vi "AskListName.vi"(1 "Default name":string, 5 "error in (no error)":errorcluster) -> (17 "List":string, 18 "OK":bool, 19 "error out":errorcluster)   [LabVIEW 2022 SP3]
doc: "Displays a standard dialog box that prompts users to enter information, such as a user name and password.\n--------------------\n\nThis Express VI is configured as follows:\n\nMessage to Display to the User:Enter the name of the new list.\nThe inputs are: \nText Entry Box: List"
uses:
  <vilib>/Utility/miscctls.llb/LVSelectionTypeDef.ctl
panel:
  in  "List":string
  out "String":string="Enter the name of the new list."
  in  "Cancel":bool
  in  "OK2":bool
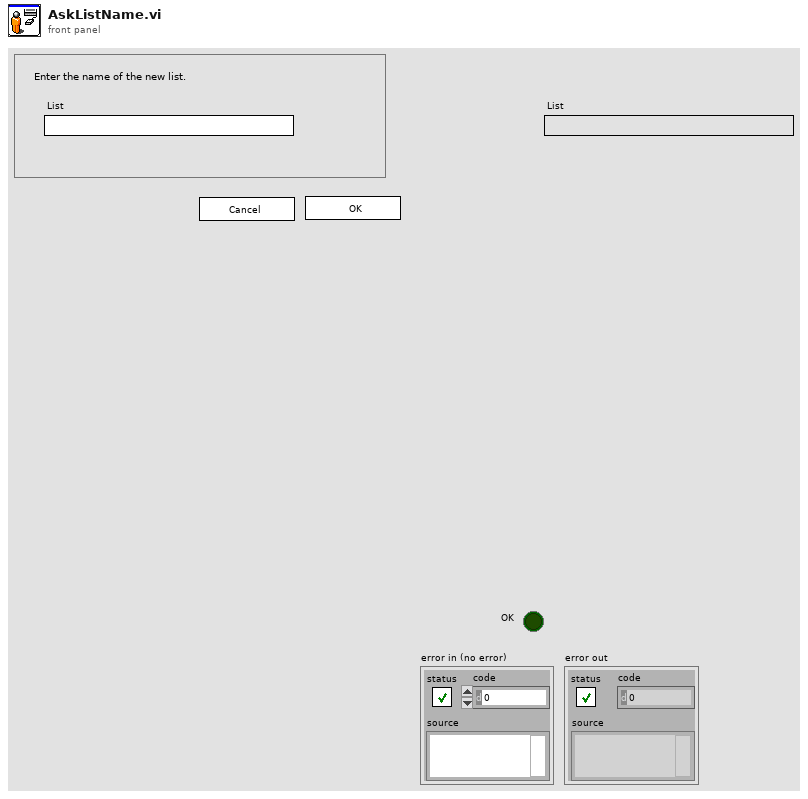
[diagram p1: front panel]
types:
  T1 = typedef "LVSelectionTypeDef.ctl" = cluster{"Selection Start":u32, "Selection End":u32}
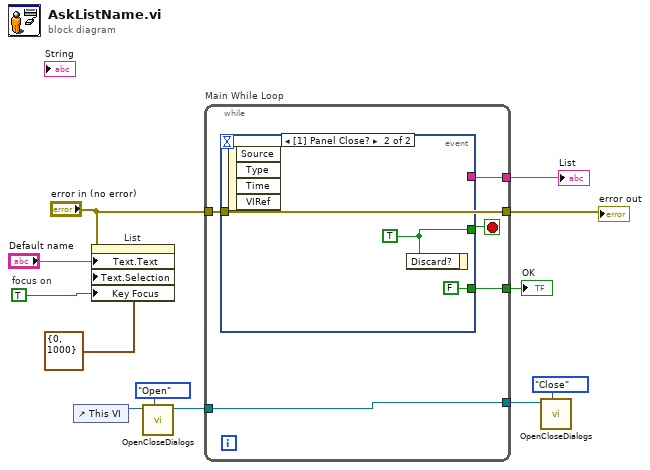
[diagram p0: block diagram]
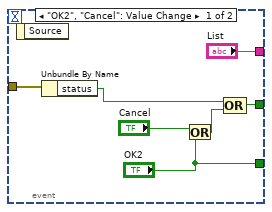
[diagram p2: hidden frame]
diagram:
  w10 = TRUE  # focus on
  n1 = control-ref of="This VI"() -> (w6:refnum<vi>)
  n2 = property on="List" class="Str"(error in="error in (no error)", "Text.Text"="Default name", "Text.Selection"=T1 {"Selection Start"=0, "Selection End"=1000}, "Key Focus"=w10) -> ()  [unwired: 1 in, 2 out]
  n3 = call "OpenCloseDialogs.vi"("Task"=enum16{"Open", "Close"}."Open", "VI in"=w6) -> ("VI out"=w3:refnum<vi>)  [unwired: 8 in, 1 out]
  n4 = while "Main While Loop" {
    tunnel: [w17] -> w12
    tunnel: "error in (no error)" -> [w16]
    tunnel: [w16] -> w2
    tunnel: [w14] -> w11
    tunnel: [w13] -> w4
    tunnel: w3 -> [w13]
    stop <- w15 stop-if-true
    n5 = event shown="[1] Panel Close?" {
      selector: _ -> [_ _]
      dyn-events: _ -> [_ _]
      timeout: _ -> [_ _]
      tunnel: ["OK2" FALSE ("OK2")] -> w17
      tunnel: [w23 w26] -> w15
      tunnel: w16 -> [w22 _]
      tunnel: ["List" _] -> w14
      event "OK2", "Cancel": Value Change {
        n6 = event-data() -> ()  [unwired: 1 in, 1 out]
        n7 = Unbundle By Name(w22) -> ("status"=w20:bool)
        n8 = Or(x="Cancel", y="OK2") -> (x .or. y?=w21:bool)
        n9 = Compound Arithmetic op=OR(w20, w21) -> (w23:bool)
      }
      event Panel Close? {
        w26 = TRUE ("Discard?")
        n10 = event-data() -> ()  [unwired: 1 in, 4 out]
        n11 = event-data("Discard?"=w26) -> ()  [unwired: 1 in, 1 out]
      }
    }
  }
  "OK" <- w12
  "error out" <- w2
  "List" <- w11
  n12 = call "OpenCloseDialogs.vi"("Task"=enum16{"Open", "Close"}."Close", "VI in"=w4) -> ()  [unwired: 8 in, 2 out]
